vi "LoggerSetDefault.vi"(8 "error in (no error)":errorcluster, 11 "LoggingActor in":refnum<class "LoggingActor.lvclass">) -> (0 "error out":errorcluster, 3 "LoggingActor out":refnum<class "LoggingActor.lvclass">)   [LabVIEW 2022 SP3, in "LoggingActor.lvlib" / "LoggingActor.lvclass"]
uses:
  LoggingActor.lvclass
  LoggingActor.lvclass/LoggingActor.ctl
  Logger/Source/Logger/_Level.ctl
  Logger/Source/Logger/Logger.lvclass
  DateTime/Source/DateTime.lvlib
  Logger/Source/Handler/Handler.lvclass
  C:/Program Files (x86)/National Instruments/LabVIEW 2022/vi.lib/ActorFramework/Actor/Actor.lvclass
  C:/Users/jakub/repos/gh/sw4sys/lv-logging-actor/LoggingActor/Source/LoggingActor/LoggingActor/LoggingActor.lvclass
  Logger/Source/FileHandler/FileHandler.lvclass
  C:/Users/jakub/repos/gh/sw4sys/lv-logging-actor/Logger/Source/Handler/Handler.lvclass
  C:/Users/jakub/repos/gh/sw4sys/lv-logging-actor/Logger/Source/FileHandler/FileHandler.lvclass
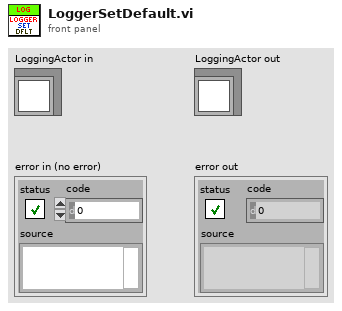
[diagram p1: front panel]
types:
  T1 = typedef "Logger.lvlib/Logger.lvclass/_Level.ctl" = enum16{"NOTSET", "DEBUG", "INFO", "WARNING", "ERROR", "CRITICAL"}
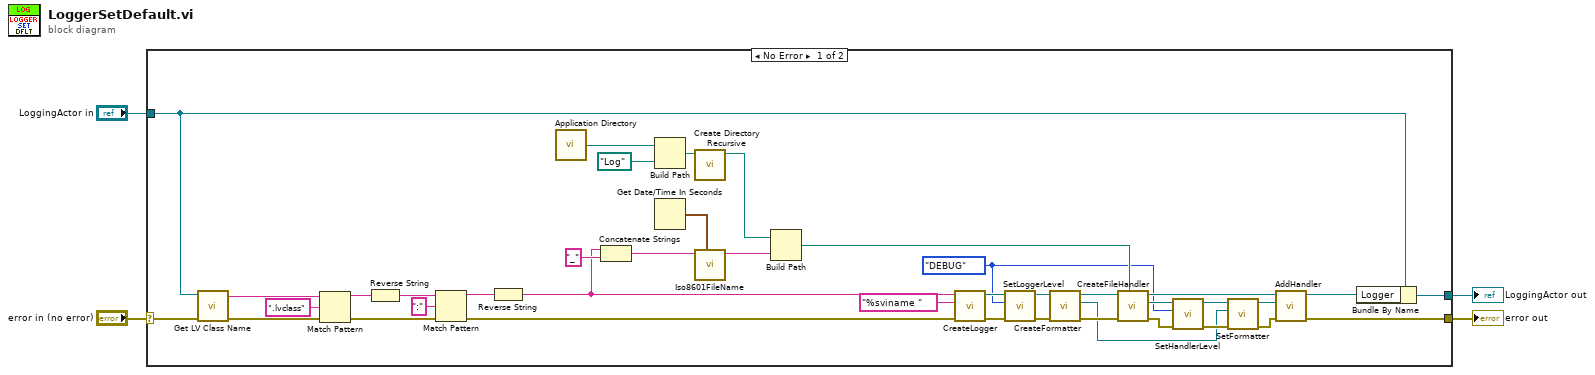
[diagram p0: block diagram]
diagram:
  n1 = case shown="No Error" "error in (no error)" {
    selector: "error in (no error)" -> [w8 w44]
    tunnel: [w7 w44] -> w3
    tunnel: [w10 w43] -> w1
    tunnel: "LoggingActor in" -> [w9 w43]
    frame No Error {
      w18 = _Level."DEBUG" ("Level")
      n2 = call <vilib>:"Get LV Class Name.vi"("error in (no error)"=w8, "object"=w9) -> ("error out"=w41:errorcluster, "class name"=w14:string)  [unwired: 8 in]
      n3 = Match Pattern(string=w14, regular expression=".lvclass") -> (before substring=w16:string)  [unwired: 1 in, 3 out]
      n4 = Reverse String(1:w16) -> (0:w13:string)
      n5 = Match Pattern(string=w13, regular expression=":") -> (before substring=w12:string)  [unwired: 1 in, 3 out]
      n6 = Reverse String(1:w12) -> (0:w11:string)
      n7 = call <vilib>:"Application Directory.vi"() -> ("Application Directory"=w38:path)
      n8 = Concatenate Strings(w11, "_" ("Prefix ('')")) -> (w31:string)
      n9 = Build Path(base path=w38, name or relative path=path "Log") -> (appended path=w36:path)
      n10 = Get Date/Time In Seconds() -> (seconds since 1Jan1904=w34:timestamp)
      n11 = call <vilib>:"Create Directory Recursive.vi"("directory"=w36) -> ("directory copy"=w33:path)  [unwired: 4 in, 2 out]
      n12 = call "Iso8601FileName.vi"("TimeStamp"=w34, "Prefix ('')"=w31) -> ("FileName"=w35:string)  [unwired: 9 in]
      n13 = Build Path(base path=w33, name or relative path=w35) -> (appended path=w30:path)
      n14 = call "CreateLogger.vi"("error in (no error)"=w41, "MessagePrefixFormat"="%sviname ", "Name"=w11) -> ("error out"=w42:errorcluster, "Logger"=w39:refnum<class "Logger.lvclass">)  [unwired: 7 in]
      n15 = call-dynamic "SetLoggerLevel.vi"("error in (no error)"=w42, "Level"=w18, "Logger in"=w39) -> ("error out"=w40:errorcluster, "Logger out"=w24:refnum<class "Logger.lvclass">)  [unwired: 7 in]
      n16 = call-dynamic "CreateFormatter.vi"("error in (no error)"=w40, "Logger in"=w24) -> ("error out"=w25:errorcluster, "Formatter"=w6:refnum<class "Formatter.lvclass">, "Logger out"=w23:refnum<class "Logger.lvclass">)  [unwired: 7 in]
      n17 = call-dynamic "CreateFileHandler.vi"("FIlePath"=w30, "error in (no error)"=w25, "Logger in"=w23) -> ("error out"=w27:errorcluster, "FileHandler"=w29:refnum<class "FileHandler.lvclass">, "Logger out"=w22:refnum<class "Logger.lvclass">)  [unwired: 6 in]
      n18 = call "SetHandlerLevel.vi"("error in (no error)"=w27, "Level"=w18, "Handler in"=w29) -> ("error out"=w26:errorcluster, "Handler out"=w28:refnum<class "Handler.lvclass">)  [unwired: 7 in]
      n19 = call "SetFormatter.vi"("error in (no error)"=w26, "Formatter in"=w6, "Handler in"=w28) -> ("error out"=w19:errorcluster, "Handler out"=w20:refnum<class "Handler.lvclass">)  [unwired: 6 in, 1 out]
      n20 = call-dynamic "AddHandler.vi"("error in (no error)"=w19, "Handler in"=w20, "Logger in"=w22) -> ("error out"=w7:errorcluster, "Logger out"=w21:refnum<class "Logger.lvclass">)  [unwired: 6 in, 1 out]
      n21 = Bundle By Name(cluster=w9, "Logger"=w21) -> (w10:refnum<class "LoggingActor.lvclass">)
    }
    frame Error {
    }
  }
  "error out" <- w3
  "LoggingActor out" <- w1
